vi "R30-realtime.vi"() -> ()   [LabVIEW 2015]
uses:
  <vilib>/rvi/interface/nirviOpenFPGA/nirviOpenFPGA.xnode
  <vilib>/rvi/interface/nirviReadWriteControl/nirviReadWriteControl.xnode
  <vilib>/functionblocks/FB Property/FB Overlay DBL.ctl
  <vilib>/functionblocks/FB Core/FB Core.xnode
  <vilib>/Instr/_visa.llb/VISA Configure Serial Port (Instr).vi
  <vilib>/Utility/error.llb/Error Cluster From Error Code.vi
  <vilib>/rvi/errors/niLvFpgaAdjustHostInterfaceError.vi
  NiFpgaLv.dll
  <vilib>/functionblocks/Control/PID/PID.vi
  <vilib>/functionblocks/NI_FunctionBlock Libraries.lvlib
  R30-Fpga.vi
  FPGA Bitfiles/Controlsoftware2_FPGATarget5_R30-Fpga_Orl9RM4cmXk.lvbitx
  <vilib>/FPGAPlugInAG/cRIO-9074/niLvFpga_Open_cRIO-9074.vi
panel:
  out "Switch magnet field set":dbl
  in  "proportional gain (Kc)":dbl=10.0
  in  "integral time (Ti, min)":dbl=0.01
  in  "derivative time (Td, min)":dbl=0.01
  out "error out 3":errorcluster
  out "error out 4":errorcluster
  out "x*y":dbl
  out "error out 7":errorcluster
  out "match + rest of string":string
  out "Switch object tesla meter":u8[](array[numeric])
  out "error out 2":errorcluster
  out "Switch object tesla meter 2":u8[](array[numeric])
  out "error out":errorcluster
  out "error out 6":errorcluster
  out "error out 8":errorcluster
  in  "Tab Control":enum32{"Page 1", "Page 2"}(tab)
  out "string":string
  out "Switch magnet field read":dbl
  out "switch magnet field":dbl(graph)
  out "Ymagnet I":fxp<+/-,26,5> format="%.3g"
  out "Y magnet v":fxp<+/-,26,5> format="%.3g"
  out "X-I":fxp<+/-,26,5> format="%.3g"
  out "X- V":fxp<+/-,26,5> format="%.3g"
  out "X+ I":fxp<+/-,26,5> format="%.3g"
  out "X+ V":fxp<+/-,26,5> format="%.3g"
  out "R30 Quad B I":fxp<+/-,26,5> format="%.3g"
  out "R30 Quad A I":fxp<+/-,26,5> format="%.3g"
  out "ESA I":fxp<+/-,26,5> format="%.3g"
  out "ESA V":fxp<+/-,26,5> format="%.3g"
  out "Y-I":fxp<+/-,26,5> format="%.3g"
  out "Y-V":fxp<+/-,26,5> format="%.3g"
  out "Y+I":fxp<+/-,26,5> format="%.3g"
  out "Y+ V":fxp<+/-,26,5> format="%.3g"
  out "R30 Y Steerer":dbl
  out "HE Y+ (1)":dbl
  out "HE Y- (1)":dbl
  out "HE X+ (1)":dbl
  out "HE X- (1)":dbl
  out "HE Quad B":dbl
  out "HE Quad A":dbl
  out "ESA":dbl
  out "Analog input":fxp<+/-,26,5>[](array[numeric]) format="%.23g"
  out "analog output":fxp<+/-,64,32>[](array[numeric]) format="%.42g"
  out "Switch magnet AP 2":bool
  out "Switch magnet FC 2":bool
  out "Detector AP 2":bool
  out "Detector FC 2":bool
  out "Switch magnet FC IN 2":bool
  out "Switch magnet FC OUT 2":bool
  out "Detector FC OUT 2":bool
  out "Detector  FC IN 2":bool
  out "Det Ap IN 2":bool
  out "Det Ap OUT 2":bool
  out "Switch Ap OUT2 2":bool
  out "Switch Ap IN 2":bool
  out "error out 5":errorcluster
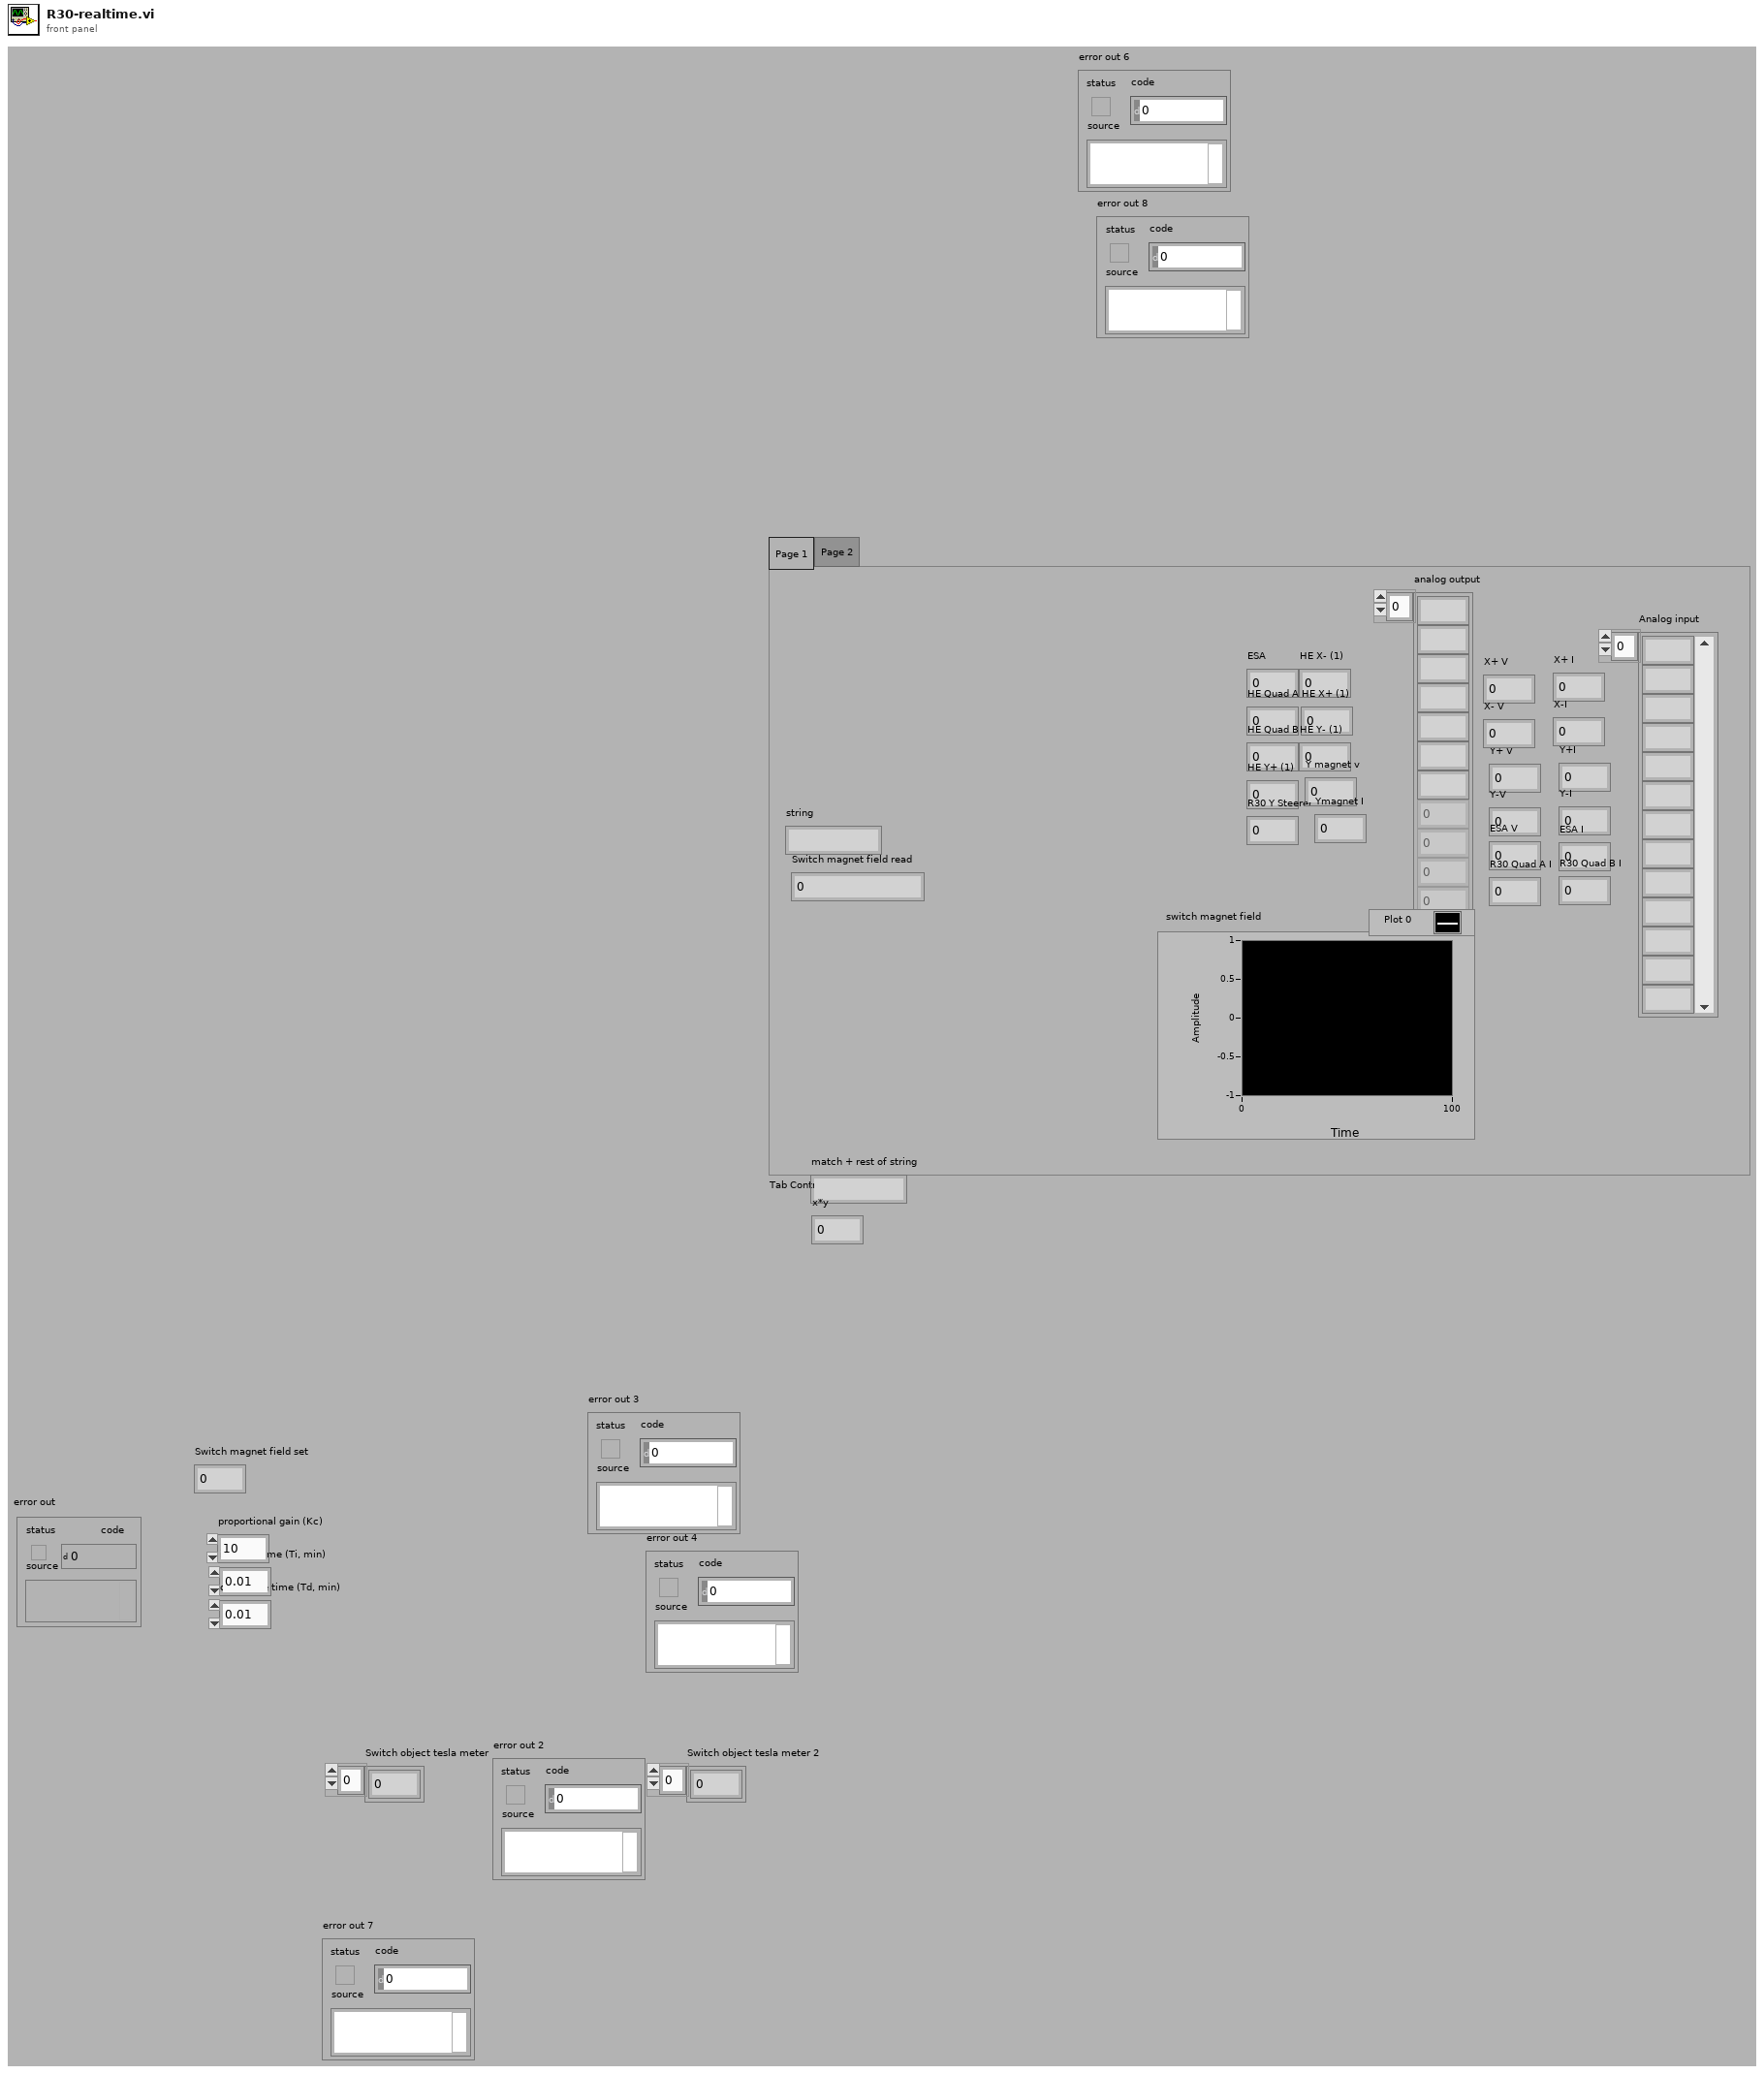
[diagram p1: front panel]
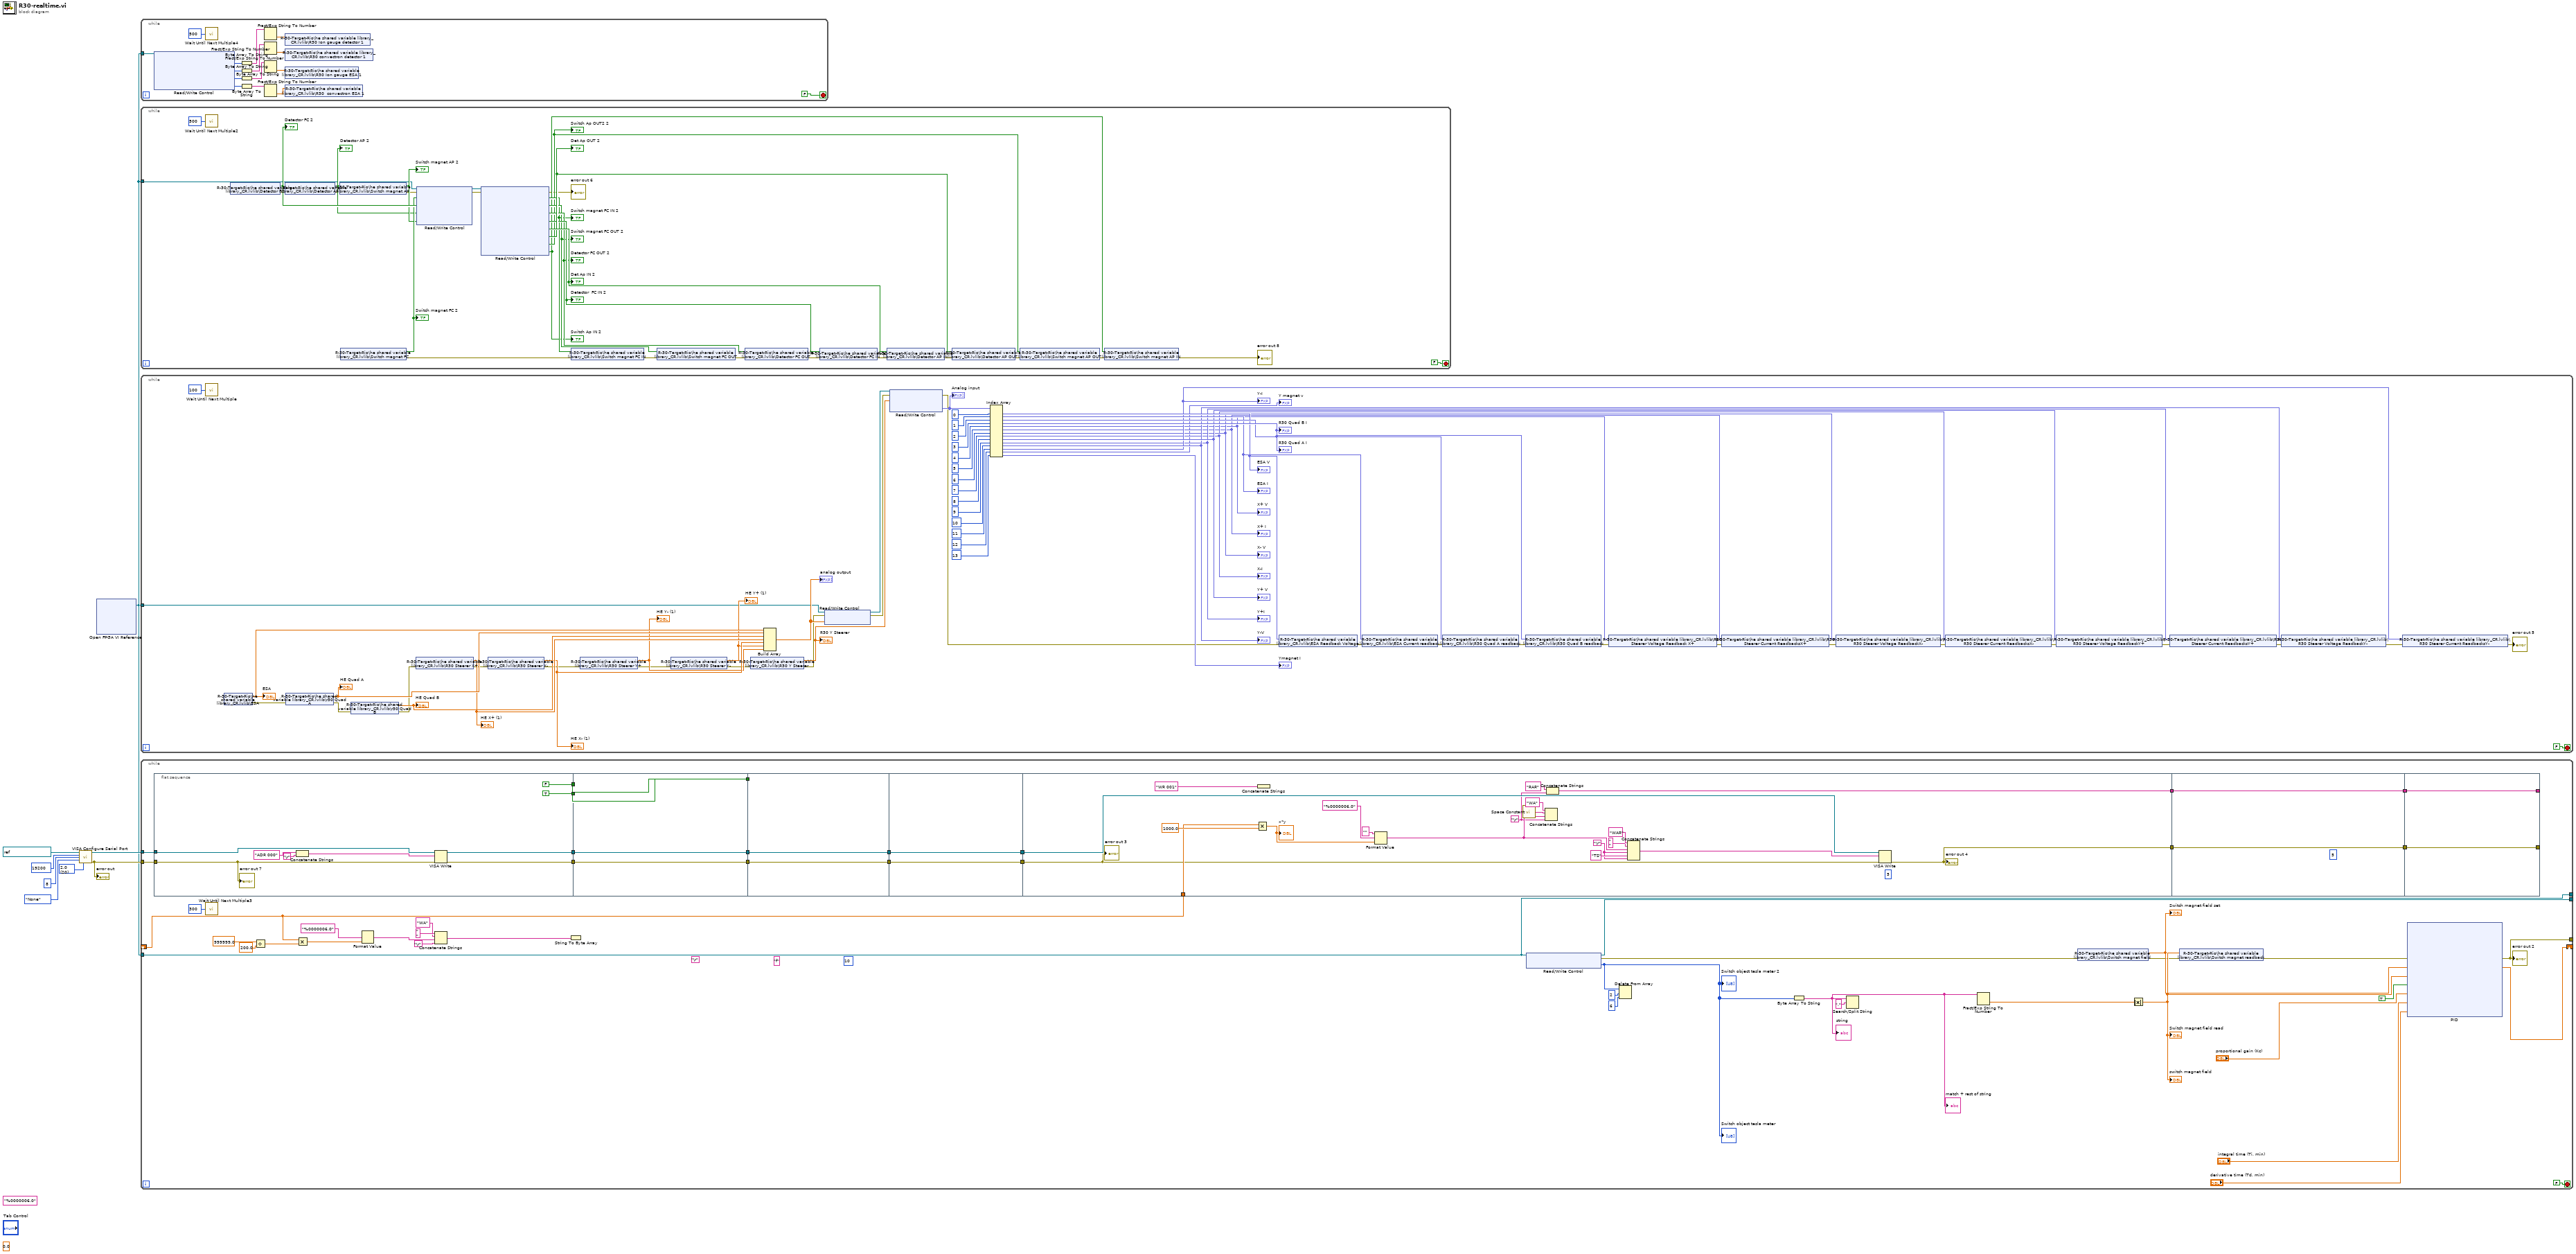
[diagram p0: block diagram]
diagram:
  w4 = u16 20 items=["1.0"=10, "1.5"=15, "2.0"=20] ("stop bits (10: 1 bit)")
  (unwired) 0.0 ("output")
  (unwired) "%0000006.0" ("format string")
  n1 = call-poly "VISA Configure Serial Port"("VISA resource name"=refnum<visa-resource-name> "ASRL1::INSTR", "baud rate (9600)"=u32 19200, "data bits (8)"=u16 8, "parity (0:none)"=enum16{"None", "Odd", "Even", "Mark", "Space"}."None", "stop bits (10: 1 bit)"=w4) -> ("VISA resource name out"=w3:refnum<visa-resource-name>, "error out"=w2:errorcluster)  [unwired: 9 in]
  "error out" <- w2
  n2 = xnode "Open FPGA VI Reference"() -> ("FPGA VI Reference Out"=w1:refnum<k20>)  [unwired: 2 in, 1 out]
  n3 = while {
    tunnel: w1 -> [w23]
    stop <- FALSE stop-if-true
    n4 = xnode "Read/Write Control"("FPGA VI Reference In"=w23) -> ("R30 Detector Ion gauge 1"=w17:u8[], "R30 Detector Convectron  1"=w18:u8[], "R30 ESA Ion gauge 1"=w19:u8[], "R30 ESA Convectron  1"=w20:u8[])  [unwired: 1 in, 2 out]
    n5 = call "Wait Until Next Multiple4"("Count(mSec)"=u32 500 ("Count(uSec)")) -> ()  [unwired: 1 out]
    n6 = Byte Array To String(unsigned byte array=w17) -> (string=w13:string)
    n7 = Byte Array To String(unsigned byte array=w18) -> (string=w14:string)
    n8 = Byte Array To String(unsigned byte array=w19) -> (string=w15:string)
    n9 = Byte Array To String(unsigned byte array=w20) -> (string=w16:string)
    n10 = Fract/Exp String To Number(string=w13) -> (number=w10:dbl)  [unwired: 3 in, 1 out]
    n11 = Fract/Exp String To Number(string=w14) -> (number=w9:dbl)  [unwired: 3 in, 1 out]
    n12 = Fract/Exp String To Number(string=w15) -> (number=w12:dbl)  [unwired: 3 in, 1 out]
    n13 = Fract/Exp String To Number(string=w16) -> (number=w11:dbl)  [unwired: 3 in, 1 out]
    n14 = shared-variable "R-30-Target-Rio\\he shared variable library_CR.lvlib\\R30 Ion gauge detector 1"(w10) -> ()  [unwired: 1 in, 1 out]
    n15 = shared-variable "R-30-Target-Rio\\he shared variable library_CR.lvlib\\R30 convectron detector 1"(w9) -> ()  [unwired: 1 in, 1 out]
    n16 = shared-variable "R-30-Target-Rio\\he shared variable library_CR.lvlib\\R30 Ion gauge ESA 1"(w12) -> ()  [unwired: 1 in, 1 out]
    n17 = shared-variable "R-30-Target-Rio\\he shared variable library_CR.lvlib\\R30  convectron ESA 1"(w11) -> ()  [unwired: 1 in, 1 out]
  }
  n18 = while {
    tunnel: w1 -> [w24]
    stop <- FALSE stop-if-true
    n19 = call "Wait Until Next Multiple2"("Count(mSec)"=u32 500 ("Count(uSec)")) -> ()  [unwired: 1 out]
    n20 = shared-variable "R-30-Target-Rio\\he shared variable library_CR.lvlib\\Detector FC"() -> (w50:bool, error out=w28:errorcluster)  [unwired: 1 in]
    "Detector FC 2" <- w50
    n21 = shared-variable "R-30-Target-Rio\\he shared variable library_CR.lvlib\\Detector AP"(error in=w28) -> (w47:bool, error out=w27:errorcluster)
    "Detector AP 2" <- w47
    n22 = shared-variable "R-30-Target-Rio\\he shared variable library_CR.lvlib\\Switch magnet AP"(error in=w27) -> (w48:bool, error out=w26:errorcluster)
    "Switch magnet AP 2" <- w48
    n23 = shared-variable "R-30-Target-Rio\\he shared variable library_CR.lvlib\\Switch magnet FC"() -> (w49:bool, error out=w36:errorcluster)  [unwired: 1 in]
    "Switch magnet FC 2" <- w49
    n24 = xnode "Read/Write Control"("FPGA VI Reference In"=w24, "error in"=w26, "Switch magnet FC"=w49, "Detector FC"=w50, "Detector AP"=w47, "Switch magnet ap"=w48) -> ("FPGA VI Reference Out"=w52:refnum<k20>, "error out"=w38:errorcluster)
    n25 = xnode "Read/Write Control"("FPGA VI Reference In"=w52, "error in"=w38) -> ("error out"=→"error out 6":errorcluster, "Switch magnet FC IN"=w41:bool, "Switch magnet FC OUT"=w42:bool, "Detector FC OUT"=w43:bool, "Detector  FC IN"=w44:bool, "Det Ap IN"=w46:bool, "Det Ap OUT"=w45:bool, "Switch Ap OUT2"=w40:bool, "Switch Ap IN"=w39:bool)  [unwired: 1 out]
    "Switch magnet FC IN 2" <- w41
    "Switch magnet FC OUT 2" <- w42
    "Detector FC OUT 2" <- w43
    "Detector  FC IN 2" <- w44
    "Det Ap IN 2" <- w46
    "Det Ap OUT 2" <- w45
    "Switch Ap OUT2 2" <- w40
    "Switch Ap IN 2" <- w39
    n26 = shared-variable "R-30-Target-Rio\\he shared variable library_CR.lvlib\\Switch magnet FC IN"(w41, error in=w36) -> (error out=w35:errorcluster)
    n27 = shared-variable "R-30-Target-Rio\\he shared variable library_CR.lvlib\\Switch magnet FC OUT"(w42, error in=w35) -> (error out=w34:errorcluster)
    n28 = shared-variable "R-30-Target-Rio\\he shared variable library_CR.lvlib\\Detector FC OUT"(w43, error in=w34) -> (error out=w33:errorcluster)
    n29 = shared-variable "R-30-Target-Rio\\he shared variable library_CR.lvlib\\Detector FC IN"(w44, error in=w33) -> (error out=w32:errorcluster)
    n30 = shared-variable "R-30-Target-Rio\\he shared variable library_CR.lvlib\\Detector AP IN"(w46, error in=w32) -> (error out=w31:errorcluster)
    n31 = shared-variable "R-30-Target-Rio\\he shared variable library_CR.lvlib\\Detector AP OUT"(w45, error in=w31) -> (error out=w30:errorcluster)
    n32 = shared-variable "R-30-Target-Rio\\he shared variable library_CR.lvlib\\Switch magnet AP OUT"(w40, error in=w30) -> (error out=w29:errorcluster)
    n33 = shared-variable "R-30-Target-Rio\\he shared variable library_CR.lvlib\\Switch magnet AP IN"(w39, error in=w29) -> (error out=→"error out 8":errorcluster)
  }
  n34 = while {
    tunnel: w1 -> [w77]
    stop <- FALSE stop-if-true
    n35 = call "Wait Until Next Multiple"("Count(mSec)"=u32 100 ("Count(uSec)")) -> ()  [unwired: 1 out]
    n36 = shared-variable "R-30-Target-Rio\\he shared variable library_CR.lvlib\\ESA"() -> (w116:dbl, error out=w74:errorcluster)  [unwired: 1 in]
    "ESA" <- w116
    n37 = shared-variable "R-30-Target-Rio\\he shared variable library_CR.lvlib\\r30 Quad A"(error in=w74) -> (w115:dbl, error out=w73:errorcluster)
    "HE Quad A" <- w115
    n38 = shared-variable "R-30-Target-Rio\\he shared variable library_CR.lvlib\\r30 Quad B"(error in=w73) -> (w114:dbl, error out=w72:errorcluster)
    "HE Quad B" <- w114
    n39 = shared-variable "R-30-Target-Rio\\he shared variable library_CR.lvlib\\R30 Steerer X+"(error in=w72) -> (w113:dbl, error out=w71:errorcluster)
    "HE X+ (1)" <- w113
    n40 = shared-variable "R-30-Target-Rio\\he shared variable library_CR.lvlib\\R30 Steerer X-"(error in=w71) -> (w112:dbl, error out=w70:errorcluster)
    "HE X- (1)" <- w112
    n41 = shared-variable "R-30-Target-Rio\\he shared variable library_CR.lvlib\\R30 Steerer Y+"(error in=w70) -> (w111:dbl, error out=w69:errorcluster)
    "HE Y- (1)" <- w111
    n42 = shared-variable "R-30-Target-Rio\\he shared variable library_CR.lvlib\\R30 Steerer Y-"(error in=w69) -> (w110:dbl, error out=w68:errorcluster)
    "HE Y+ (1)" <- w110
    n43 = shared-variable "R-30-Target-Rio\\he shared variable library_CR.lvlib\\R30 Y Steerer"(error in=w68) -> (w80:dbl, error out=w67:errorcluster)
    "R30 Y Steerer" <- w80
    n44 = Build Array(w116, w115, w114, w113, w112, w110, w111) -> (w79:dbl[])
    "analog output" <- w79
    n45 = xnode "Read/Write Control"("FPGA VI Reference In"=w77, "error in"=w67, "analog output"=w79) -> ("FPGA VI Reference Out"=w109:refnum<k20>, "error out"=w75:errorcluster)
    n46 = xnode "Read/Write Control"("FPGA VI Reference In"=w109, "error in"=w75, "y steerer magnet"=w80) -> ("error out"=w66:errorcluster, "analog readback"=w76:fxp<+/-,26,5>[])  [unwired: 1 out]
    "Analog input" <- w76
    n47 = Index Array(array=w76, index #1=0 ("index"), index #2=1 ("index"), index #3=2 ("index"), index #4=3 ("index"), index #5=4 ("index"), index #6=5 ("index"), index #7=6 ("index"), index #8=7 ("index"), index #9=8 ("index"), index #10=9 ("index"), index #11=10 ("index"), index #12=11 ("index"), index #13=12 ("index"), index #14=13 ("index")) -> (element #1=w93:fxp<+/-,26,5>, element #2=w94:fxp<+/-,26,5>, element #3=w95:fxp<+/-,26,5>, element #4=w96:fxp<+/-,26,5>, element #5=w86:fxp<+/-,26,5>, element #6=w85:fxp<+/-,26,5>, element #7=w88:fxp<+/-,26,5>, element #8=w87:fxp<+/-,26,5>, element #9=w92:fxp<+/-,26,5>, element #10=w89:fxp<+/-,26,5>, element #11=w91:fxp<+/-,26,5>, element #12=w90:fxp<+/-,26,5>, element #13=→"Y magnet v":fxp<+/-,26,5>, element #14=→"Ymagnet I":fxp<+/-,26,5>)
    "Y+ V" <- w92
    "Y+I" <- w89
    "Y-V" <- w91
    "Y-I" <- w90
    "ESA V" <- w93
    "ESA I" <- w94
    "R30 Quad A I" <- w95
    "R30 Quad B I" <- w96
    "X+ V" <- w86
    "X+ I" <- w85
    "X- V" <- w88
    "X-I" <- w87
    n48 = shared-variable "R-30-Target-Rio\\he shared variable library_CR.lvlib\\ESA Readback Voltage"(w93, error in=w66) -> (error out=w65:errorcluster)
    n49 = shared-variable "R-30-Target-Rio\\he shared variable library_CR.lvlib\\ESA Current readback"(w94, error in=w65) -> (error out=w64:errorcluster)
    n50 = shared-variable "R-30-Target-Rio\\he shared variable library_CR.lvlib\\R30 Quad A readback"(w95, error in=w64) -> (error out=w63:errorcluster)
    n51 = shared-variable "R-30-Target-Rio\\he shared variable library_CR.lvlib\\R30 Quad B readback"(w96, error in=w63) -> (error out=w62:errorcluster)
    n52 = shared-variable "R-30-Target-Rio\\he shared variable library_CR.lvlib\\R30 Steerer Voltage Readback X+"(w86, error in=w62) -> (error out=w61:errorcluster)
    n53 = shared-variable "R-30-Target-Rio\\he shared variable library_CR.lvlib\\R30 Steerer Current ReadbacksX+"(w85, error in=w61) -> (error out=w60:errorcluster)
    n54 = shared-variable "R-30-Target-Rio\\he shared variable library_CR.lvlib\\R30 Steerer Voltage ReadbackX-"(w88, error in=w60) -> (error out=w59:errorcluster)
    n55 = shared-variable "R-30-Target-Rio\\he shared variable library_CR.lvlib\\R30 Steerer Current ReadbacksX-"(w87, error in=w59) -> (error out=w58:errorcluster)
    n56 = shared-variable "R-30-Target-Rio\\he shared variable library_CR.lvlib\\R30 Steerer Voltage ReadbackY+"(w92, error in=w58) -> (error out=w57:errorcluster)
    n57 = shared-variable "R-30-Target-Rio\\he shared variable library_CR.lvlib\\R30 Steerer Current ReadbacksY+"(w89, error in=w57) -> (error out=w56:errorcluster)
    n58 = shared-variable "R-30-Target-Rio\\he shared variable library_CR.lvlib\\R30 Steerer Voltage ReadbackY-"(w91, error in=w56) -> (error out=w55:errorcluster)
    n59 = shared-variable "R-30-Target-Rio\\he shared variable library_CR.lvlib\\R30 Steerer Current ReadbacksY-"(w90, error in=w55) -> (error out=→"error out 5":errorcluster)
  }
  n60 = while {
    tunnel: [w123] -> _
    tunnel: [w129] -> _
    shift-right: [w161] -> _
    shift-left: _ -> [w130]
    tunnel: [w122] -> _
    tunnel: w2 -> [w133]
    tunnel: w3 -> [w132]
    tunnel: w1 -> [w122]
    stop <- FALSE stop-if-true
    (unwired) "\r"
    (unwired) u32 10 ("byte count")
    (unwired) "f" ("write buffer")
    n61 = flat-sequence {
      tunnel: [w172] -> w149
      tunnel: [TRUE ("Communications On/Off")] -> w148
      tunnel: [FALSE ("Communications Mode")] -> w147
      tunnel: [w170] -> w146
      tunnel: w133 -> [w168]
      tunnel: w132 -> [w169]
      tunnel: w149 -> [w180]
      tunnel: [w180] -> w145
      tunnel: [w179] -> w144
      tunnel: w148 -> [w179]
      tunnel: w147 -> [w178]
      tunnel: [w178] -> w143
      tunnel: [w177] -> w142
      tunnel: w146 -> [w177]
      tunnel: w145 -> [w181]
      tunnel: w144 -> [_]
      tunnel: w143 -> [_]
      tunnel: [w181] -> w141
      tunnel: w142 -> [w182]
      tunnel: [w182] -> w140
      tunnel: w141 -> [w184]
      tunnel: [w184] -> w139
      tunnel: [w183] -> w138
      tunnel: w140 -> [w183]
      tunnel: w139 -> [w197]
      tunnel: [w191] -> w137
      tunnel: w138 -> [w186]
      tunnel: [w192] -> w136
      tunnel: w130 -> [w193]
      tunnel: w137 -> [w206]
      tunnel: [w205] -> w135
      tunnel: w136 -> [w205]
      tunnel: [w206] -> w134
      tunnel: w135 -> [w207]
      tunnel: w134 -> [w208]
      tunnel: [w208] -> _
      tunnel: [w207] -> _
      frame #0 {
        n62 = Concatenate Strings("ADR 000" ("Write String"), "\r") -> (w171:string)
        n63 = VISA Write(VISA resource name=w169, write buffer=w171, error in (no error)=w168) -> (VISA resource name out=w172:refnum<visa-resource-name>, error out=w170:errorcluster)  [unwired: 1 out]
        "error out 7" <- w168
      }
      frame #1 {
      }
      frame #2 {
      }
      frame #3 {
      }
      frame #4 {
        (unwired) u32 5 ("byte count")
        w187 = "\r"
        w200 = "\r"
        n64 = Multiply(x=w193, y=1000.0) -> (x*y=w194:dbl)
        "x*y" <- w194
        n65 = Concatenate Strings("WR 001" ("Write String")) -> ()  [unwired: 1 out]
        n66 = Format Value(string ("")="", format string="%0000006.0", value (0)=w194) -> (output string=w188:string)
        n67 = call <vilib>:"Space Constant.vi"() -> ("String"=w189:string)
        n68 = Concatenate Strings("WA" ("Write String"), w189, w188, w187) -> ()  [unwired: 1 out]
        n69 = Concatenate Strings("RAR" ("Write String"), w187) -> (w191:string)
        n70 = Concatenate Strings("WAR", " ", w188, w200, "TS" ("string"), w200) -> (w185:string)
        n71 = VISA Write(VISA resource name=w197, write buffer=w185, error in (no error)=w186) -> (error out=w192:errorcluster)  [unwired: 2 out]
        "error out 4" <- w192
        "error out 3" <- w186
      }
      frame #5 {
        (unwired) u32 5 ("byte count")
      }
      frame #6 {
      }
    }
    n72 = call "Wait Until Next Multiple3"("Count(mSec)"=u32 300 ("millisecond multiple")) -> ()  [unwired: 1 out]
    n73 = Divide(x=999999.0, y=200.0) -> (x/y=w165:dbl)
    n74 = Multiply(x=w130, y=w165) -> (x*y=w131:dbl)
    n75 = Format Value(format string="%0000006.0", value (0)=w131) -> (output string=w150:string)  [unwired: 1 out]
    n76 = Concatenate Strings("WA", " ", w150, "\r") -> (w152:string)
    n77 = String To Byte Array(string=w152) -> ()  [unwired: 1 out]
    n78 = xnode "Read/Write Control"("FPGA VI Reference In"=w122) -> ("FPGA VI Reference Out"=w129:refnum<k20>, "error out"=w126:errorcluster, "Switch object tesla meter"=w121:u8[])  [unwired: 1 in]
    "Switch object tesla meter" <- w121
    "Switch object tesla meter 2" <- w121
    n79 = Delete From Array(array=w121, length=2, index=6) -> ()  [unwired: 2 out]
    n80 = Byte Array To String(unsigned byte array=w121) -> (string=w118:string)
    "string" <- w118
    "match + rest of string" <- w118
    n81 = Search/Split String(string=w118, search string/char (-)=".") -> ()  [unwired: 4 out]
    n82 = Fract/Exp String To Number(string=w118) -> (number=w127:dbl)  [unwired: 3 in, 1 out]
    n83 = shared-variable "R-30-Target-Rio\\he shared variable library_CR.lvlib\\Switch magnet field"(error in=w126) -> (w159:dbl, error out=w125:errorcluster)
    "Switch magnet field set" <- w159
    n84 = Absolute Value(x=w127) -> (abs(x)=w128:dbl)
    "Switch magnet field read" <- w128
    "switch magnet field" <- w128
    n85 = shared-variable "R-30-Target-Rio\\he shared variable library_CR.lvlib\\Switch magnet readback"(w128, error in=w125) -> (error out=w124:errorcluster)
    n86 = xnode "PID"("error in"=w124, "setpoint"=w159, "process variable"=w128, "auto? (T)"=TRUE, "proportional gain (Kc)"="proportional gain (Kc)", "integral time (Ti, min)"="integral time (Ti, min)", "derivative time (Td, min)"="derivative time (Td, min)") -> ("error out"=w123:errorcluster, "output"=w161:dbl)
    "error out 2" <- w123
  }
